vi "Measurement UI.vi"() -> ()   [LabVIEW 2024, in "PMIC_Efficiency.lvlib"]
uses:
  PMIC_Efficiency.lvlib
panel:
  in  "Argus Configuration":enum32{"Settings", "Page 2"}(tab)
  in  "Source current limit (A)":dbl=25.0
  in  "Source power boundary (W)":dbl=300.0
  in  "Source values (V)":dbl[](array[numeric])
  in  "Source resource device name":refnum<k15> caption="Source device name"
  in  "Load voltage limit (V)":dbl=6.0
  in  "Load source device name":refnum<k15> caption="Load device name"
  in  "Source delay (s)":dbl=0.005
  in  "Current load level stop":dbl=24.0 min=0.0 step=0.1
  in  "Current load level start":dbl=0.1 min=0.0 step=0.1
  in  "Points or Points/Decade":i32=10
  in  "Sweep type":u32(ring)=1 items=["Linear", "Logarithmic"]
  in  "Timeout (s)":dbl=15.0 format="%.3p"
  in  "Aperture time (s)":dbl=0.005
  in  "DUT setup time (s)":dbl=1.0 format="%.2p"
  in  "Source device name":string="PXIe-4151"
  in  "Load device name":string="PXIe-4051"
  out "Load currents":dbl[](array[numeric])
  out "Efficiency (%)":dbl[](array[numeric])
  out "Load current points":i32
  out "DUT Efficiency (%) vs. Load Current (A)":cluster{dbl[], dbl[]}[](graph) caption="Current (Amps) vs Voltage (Volts)"
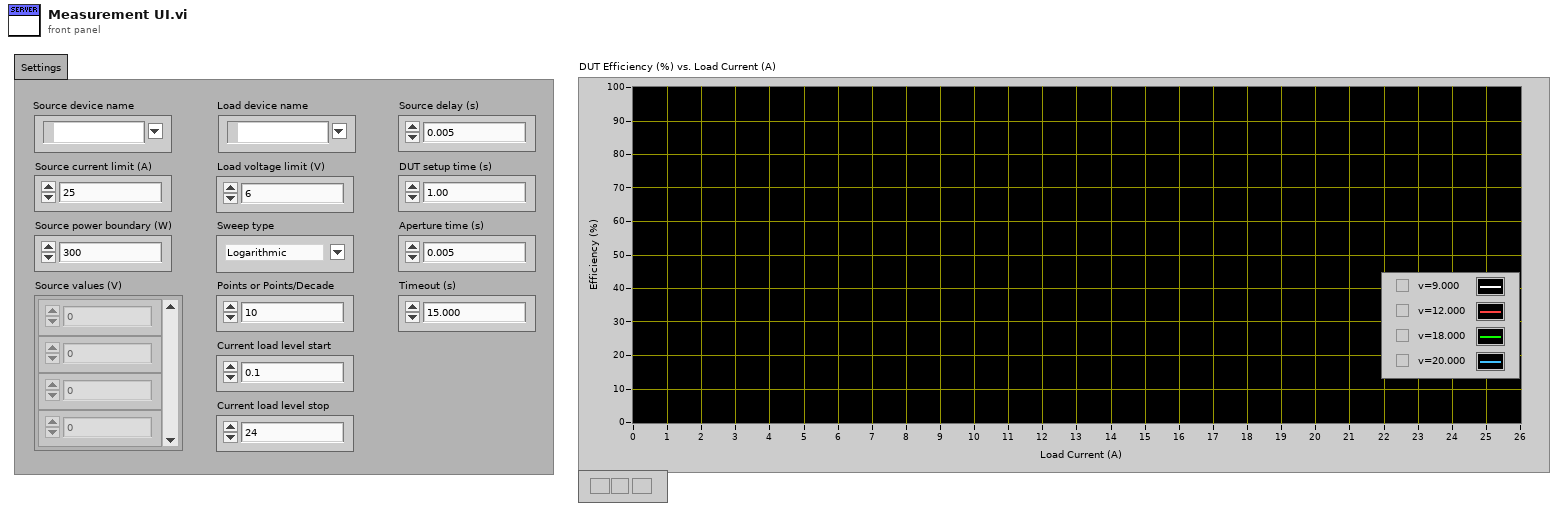
[diagram p1: front panel]
types:
  T1 = cluster{"Load currents":dbl[], "Efficiency (%)":dbl[]}
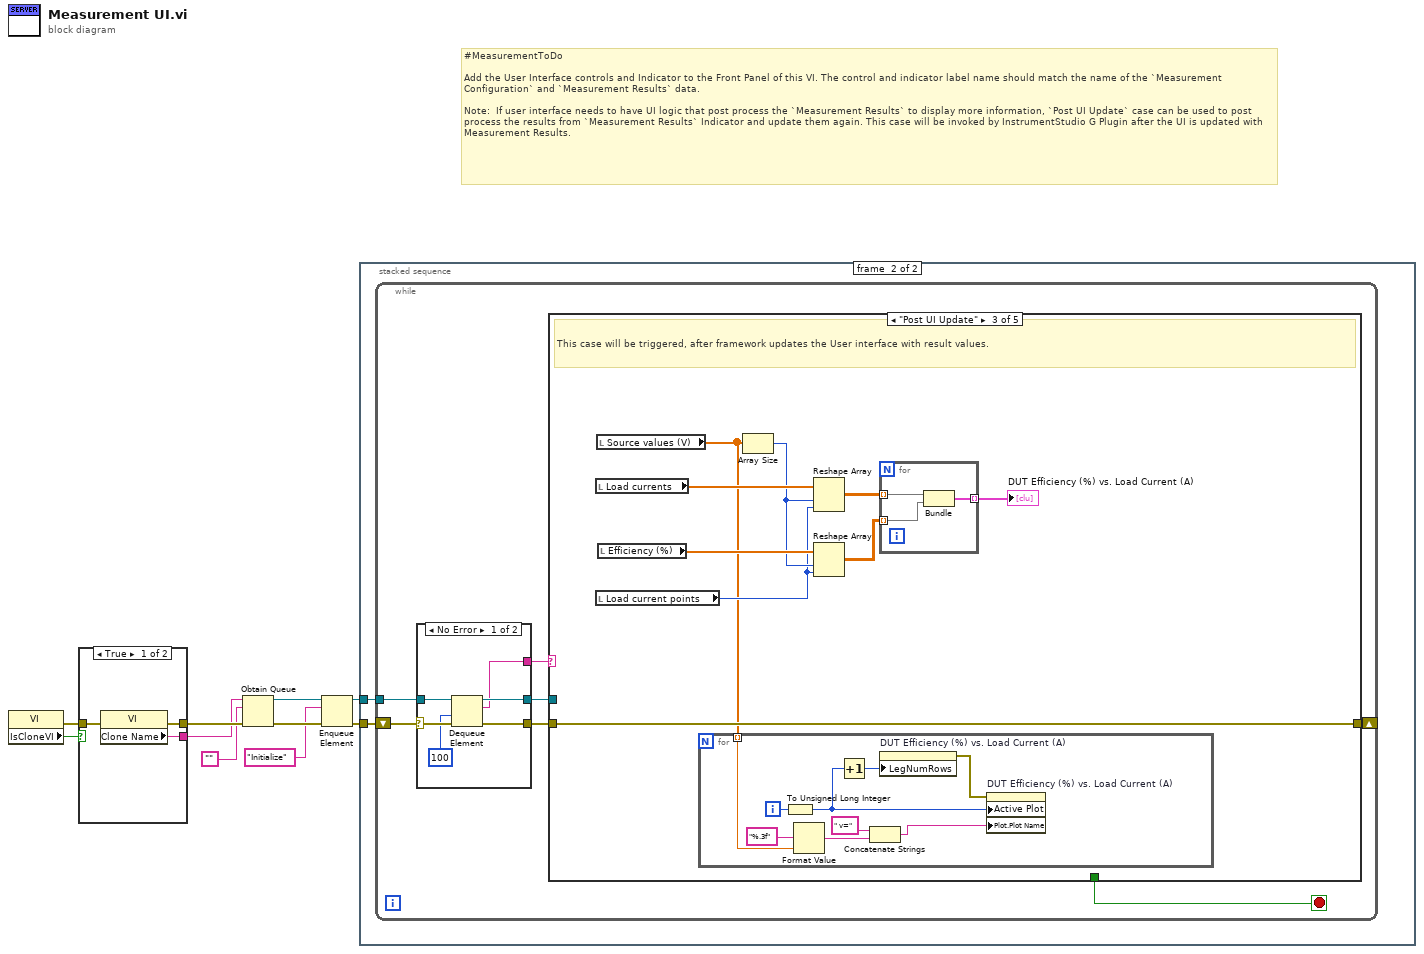
[diagram p0: block diagram]
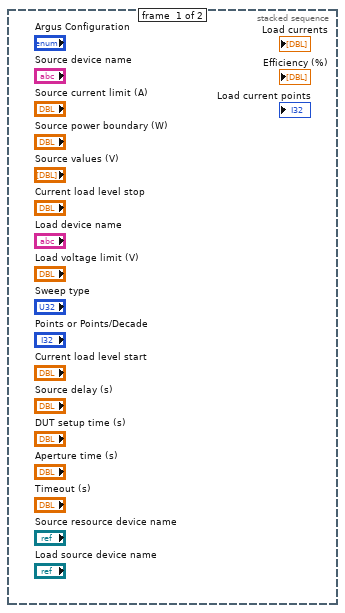
[diagram p2: hidden frame]
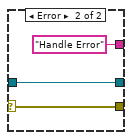
[diagram p3: hidden frame]
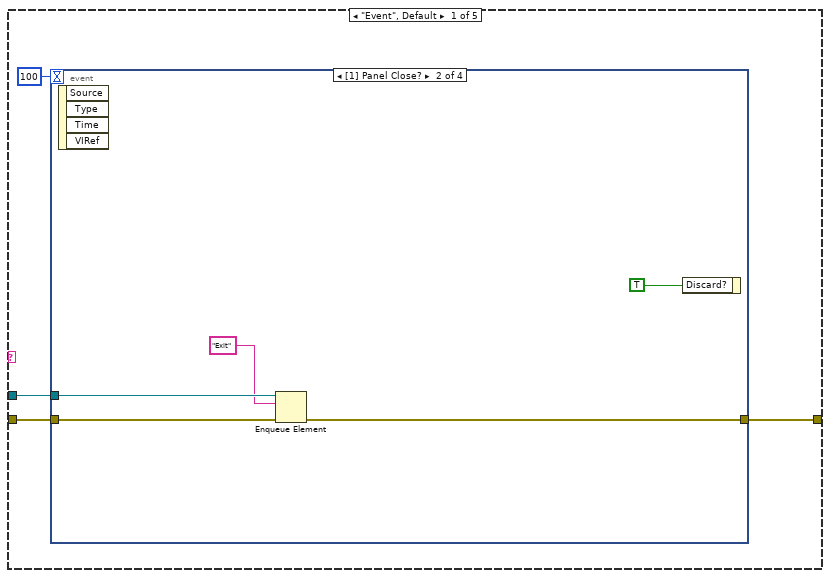
[diagram p4: hidden frame]
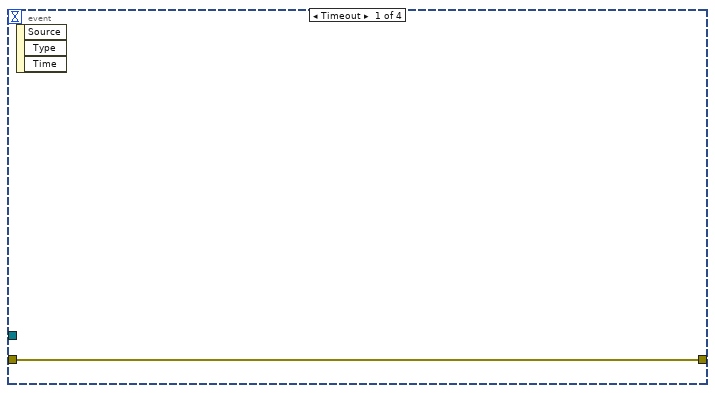
[diagram p5: hidden frame]
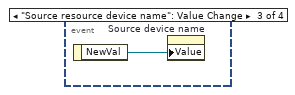
[diagram p6: hidden frame]
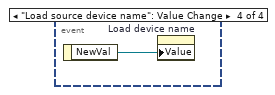
[diagram p7: hidden frame]
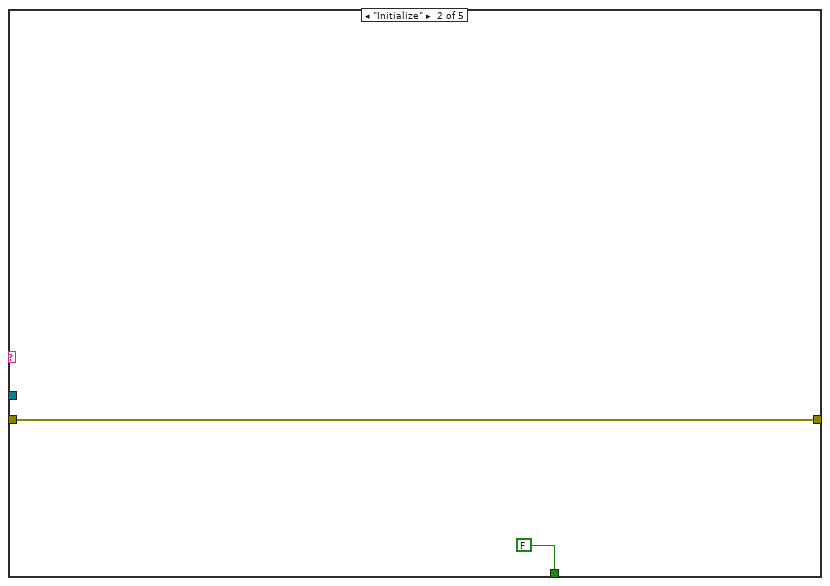
[diagram p8: hidden frame]
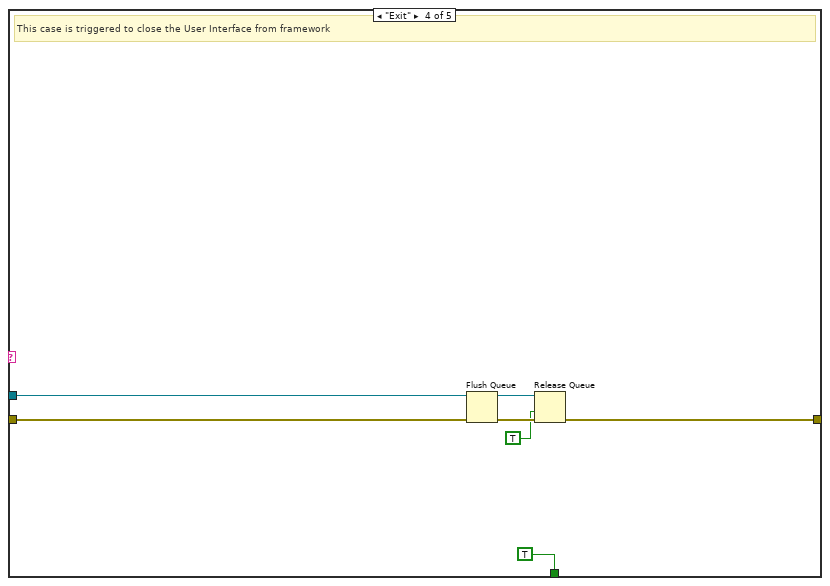
[diagram p9: hidden frame]
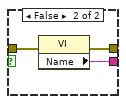
[diagram p11: hidden frame]
diagram:
  # "#MeasurementToDo  \n\nAdd the User Interface controls and Indicator to the Front Panel of this VI. The control and indicator label name should match the name of the `Measurement Configuration` and `Measurement Results` data.\n\nNote:  If user interface needs to have UI logic that post process the `Measurement Results` to display more information, `Post UI Update` case can be used to post process the results from `Measurement Results` Indicator and update them again. This case will be invoked by InstrumentStudio G Plugin after the UI is updated with Measurement Results."
  n1 = property class="VI"() -> (error out=w1:errorcluster, "IsCloneVI"=w2:bool)  [unwired: 2 in, 1 out]
  n2 = case shown="True" w2 {
    tunnel: [w13 w16] -> w10
    tunnel: [w12 w15] -> w9
    tunnel: w1 -> [w11 w14]
    frame True {
      n3 = property class="VI"(error in=w11) -> (error out=w13:errorcluster, "Clone Name"=w12:string)  [unwired: 1 in, 1 out]
    }
    frame False {
      n4 = property class="VI"(error in=w14) -> (error out=w16:errorcluster, "Name"=w15:string)  [unwired: 1 in, 1 out]
    }
  }
  n5 = Obtain Queue(name (unnamed)=w9, element data type="", error in (no error)=w10) -> (queue out=w6:refnum<queue>, error out=w8:errorcluster)  [unwired: 2 in, 1 out]
  n6 = Enqueue Element(queue=w6, element="Initialize", error in (no error)=w8) -> (queue out=w5:refnum<queue>, error out=w7:errorcluster)  [unwired: 1 in, 1 out]
  n7 = stacked-sequence {
    tunnel: w7 -> [_ w18]
    tunnel: w5 -> [_ w17]
    frame #0 {
    }
    frame #1 {
      n8 = while {
        shift-right: [w20] -> _
        shift-left: w18 -> [w25]
        tunnel: w17 -> [w23]
        stop <- w19 stop-if-true
        n9 = case shown="No Error" w25 {
          selector: w25 -> [w31 w34]
          tunnel: [w30 w34] -> w24
          tunnel: w23 -> [w29 w33]
          tunnel: [w28 w33] -> w22
          tunnel: [w27 "Handle Error"] -> w21
          frame No Error {
            n10 = Dequeue Element(queue=w29, timeout in ms (-1)=100, error in (no error)=w31) -> (queue out=w28:refnum<queue>, element=w27:string, error out=w30:errorcluster)  [unwired: 1 out]
          }
          frame Error {
          }
        }
        n11 = case shown="\"Post UI Update\"" w21 {
          tunnel: w24 -> [w37 w48 w57 w76 w77]
          tunnel: w22 -> [w35 _ _ w74 _]
          tunnel: [w38 w48 w57 w71 w77] -> w20
          tunnel: [_ FALSE _ TRUE _] -> w19
          frame "Event", Default {
            n12 = event shown="[1] Panel Close?" {
              selector: _ -> [_ _ _ _]
              dyn-events: _ -> [_ _ _ _]
              timeout: 100 -> [_ _ _ _]
              tunnel: [w39 w42 _ _] -> w38
              tunnel: w37 -> [w39 w43 _ _]
              tunnel: w35 -> [_ w41 _ _]
              event Timeout {
                n13 = event-data() -> ()  [unwired: 1 in, 3 out]
              }
              event Panel Close? {
                n14 = event-data() -> ()  [unwired: 1 in, 4 out]
                n15 = Enqueue Element(queue=w41, element="Exit", error in (no error)=w43) -> (error out=w42:errorcluster)  [unwired: 1 in, 2 out]
                n16 = event-data("Discard?"=TRUE) -> ()  [unwired: 1 in, 1 out]
              }
              event "Source resource device name": Value Change {
                n17 = event-data() -> ("NewVal"=w45:refnum<k15>)  [unwired: 1 in]
                n18 = property on="Source device name" class="Str"("Value"=w45) -> ()  [unwired: 2 in, 2 out]
              }
              event "Load source device name": Value Change {
                n19 = event-data() -> ("NewVal"=w46:refnum<k15>)  [unwired: 1 in]
                n20 = property on="Load device name" class="Str"("Value"=w46) -> ()  [unwired: 2 in, 2 out]
              }
            }
          }
          frame "Initialize" {
          }
          frame "Post UI Update" {
            # "This case will be triggered, after framework updates the User interface with result values."
            n21 = local read "Load currents"() -> (w56:dbl[])
            n22 = local read "Load current points"() -> (w50:i32)
            n23 = local read "Source values (V)"() -> (w49:dbl[])
            n24 = local read "Efficiency (%)"() -> (w55:dbl[])
            n25 = for {
              tunnel: w49 -> [w58] mode=indexing
              i -> [w59]
              n26 = To Unsigned Long Integer(number=w59) -> (unsigned 32bit integer=w63:u32)
              n27 = Format Value(format string="%.3f", value (0)=w58) -> (output string=w64:string)  [unwired: 1 out]
              n28 = Increment(x=w63) -> (x+1=w62:u32)
              n29 = Concatenate Strings(" v=" ("string"), w64) -> (w60:string)
              n30 = property on="DUT Efficiency (%) vs. Load Current (A)" class="XYGraph (strict)"("LegNumRows"=w62) -> (error out=w61:errorcluster)  [unwired: 2 in, 1 out]
              n31 = property on="DUT Efficiency (%) vs. Load Current (A)" class="XYGraph (strict)"(error in=w61, "Active Plot"=w63, "Plot.Plot Name"=w60) -> ()  [unwired: 1 in, 2 out]
            }
            n32 = Array Size(array=w49) -> (size(s)=w54:i32)
            n33 = Reshape Array(w56, w54, w50) -> (w53:dbl[][])
            n34 = Reshape Array(w55, w54, w50) -> (w52:dbl[][])
            n35 = for {
              tunnel: w53 -> [w69] mode=indexing
              tunnel: w52 -> [w68] mode=indexing
              tunnel: [w67] -> w51 mode=indexing
              n36 = Bundle("Load currents"=w69, "Efficiency (%)"=w68) -> (w67:T1)  [unwired: 1 in]
            }
            "DUT Efficiency (%) vs. Load Current (A)" <- w51
          }
          frame "Exit" {
            # "This case is triggered to close the User Interface from framework"
            n37 = Flush Queue(queue=w74, error in (no error)=w76) -> (queue out=w73:refnum<queue>, error out=w72:errorcluster)  [unwired: 1 out]
            n38 = Release Queue(queue=w73, force destroy? (F)=TRUE, error in (no error)=w72) -> (error out=w71:errorcluster)  [unwired: 2 out]
          }
          frame "Handle Error" {
          }
        }
      }
    }
  }
